vi "Reset_Power_Supply.vi"(8 "error in (no error)":errorcluster, 11 "resource name":refnum<k15>="PSU") -> (0 "error out":errorcluster {"code" format="%.0x"})   [LabVIEW 2018]
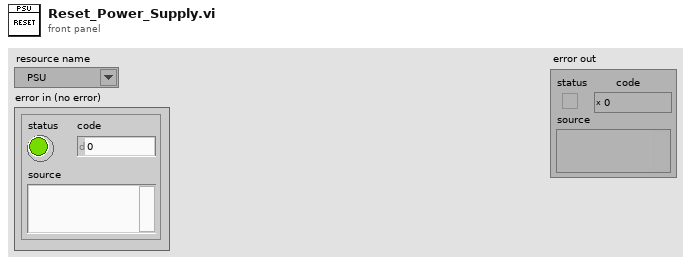
[diagram p1: front panel]
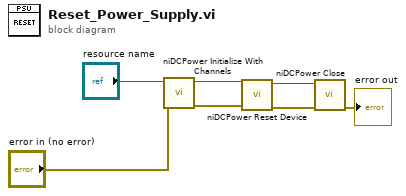
[diagram p0: block diagram]
diagram:
  n1 = call <instrlib>:"niDCPower Initialize With Channels.vi"("error in (no error)"="error in (no error)", "resource name"="resource name") -> ("error out"=w4:errorcluster, "instrument handle out"=w5:refnum<k15>)  [unwired: 2 in, 6 out]
  n2 = call <instrlib>:"niDCPower Reset Device.vi"("error in (no error)"=w4, "instrument handle"=w5) -> ("error out"=w6:errorcluster, "instrument handle out"=w7:refnum<k15>)  [unwired: 8 in]
  n3 = call <instrlib>:"niDCPower Close.vi"("error in (no error)"=w6, "instrument handle"=w7) -> ("error out"=→"error out":errorcluster)  [unwired: 9 in]
